vi "Customized FPGA Multiplier.vi"(1 "coef (24.1)":i32, 2 "multiplicand (16.8)":i16) -> (0 "product (32.9)":i32)   [LabVIEW 2023]
doc: "Customizes an integer multiplier that implements a fixed-point multiplication of 24.1 x 16.8 --> 32.9, where a fixed-point number is represented in the format of (wl.iwl)."
uses:
  <vilib>/rvi/Arithmetic/AddSubMult/XNode/nirviSatArithmetic.xnode
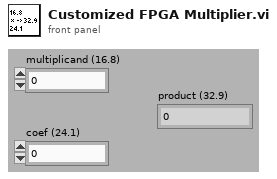
[diagram p1: front panel]
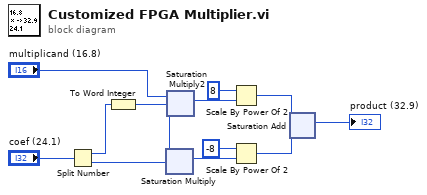
[diagram p0: block diagram]
diagram:
  n1 = Split Number(x="coef (24.1)") -> (hi(x)=w10:u16, lo(x)=w11:u16)
  n2 = To Word Integer(number=w10) -> (16bit integer=w9:i16)
  n3 = xnode ("Saturation Multiply")("x"="multiplicand (16.8)", "y"=w11) -> ("x*y"=w5:i32)
  n4 = xnode ("Saturation Multiply2")("x"="multiplicand (16.8)", "y"=w9) -> ("x*y"=w7:i32)
  n5 = Scale By Power Of 2(n=8, x=w7) -> (x*2^n=w3:i32)
  n6 = Scale By Power Of 2(n=-8, x=w5) -> (x*2^n=w2:i32)
  n7 = xnode ("Saturation Add")("x"=w3, "y"=w2) -> ("x+y"=→"product (32.9)":i32)
